vi "IonHeating.vi"(0 "Rotating Wall Parameters":T1={"Start Frequency"=20000.0, "Stop Frequency"=20000.0, "Sweep Time"=0.0, "Amplitude"=1.5, "Phase (ch.1)"=0.001, "Phase (Ch.2)"=90.0} {"Sweep Time" format="%.4f"; "Phase (Ch.2)" min=-1800.0 max=1800.0 step=0.1 format="%.3f"; "Phase (ch.1)" min=-1800.0 max=1800.0 step=0.1 format="%.3f"; "Stop Frequency" format="%#.5p"; "Start Frequency" format="%#.5p"; "Amplitude" min=0.0 max=4.0 format="%.3f"}, 1 "On/Off":bool, 2 "VISAsession":refnum<visa-resource-name>="wavefactoryU10") -> ()   [LabVIEW 2018]
panel:
  out "x-y 5":u32=300
  out "x-y 4":u32=100
  out "x-y 3":u32=901
  out "x-y 2":u32=800
  out "x-y":u32=600
  out "millisecond timer value":u32=88672931
  out "error out":errorcluster caption="Error OUT"
  # "Turn-on\nTimes (ms)"
  # "Turn-off\nTimes (ms)"
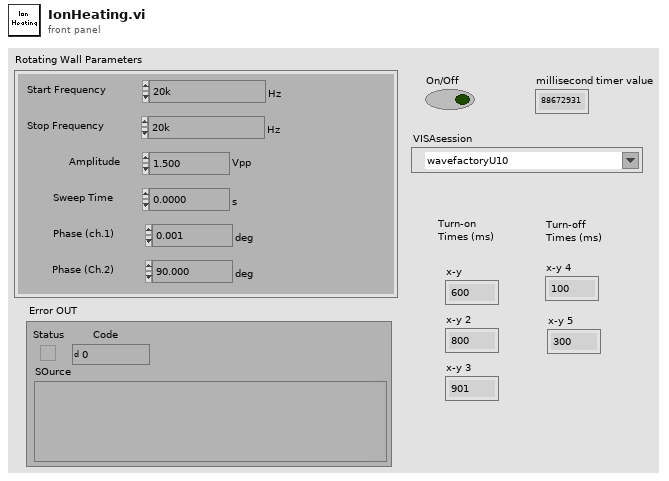
[diagram p1: front panel]
types:
  T1 = cluster{"Start Frequency":dbl, "Stop Frequency":dbl, "Sweep Time":dbl, "Amplitude":dbl, "Phase (ch.1)":dbl, "Phase (Ch.2)":dbl}
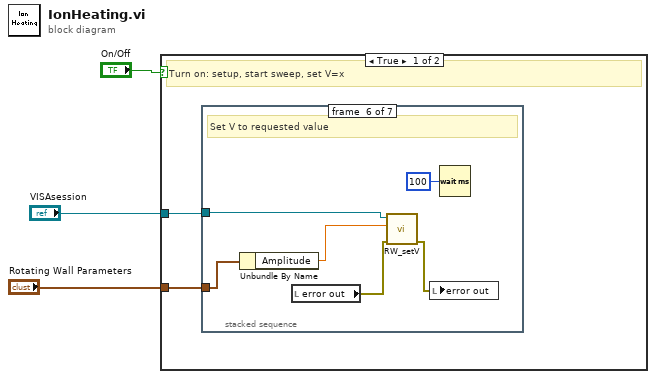
[diagram p0: block diagram]
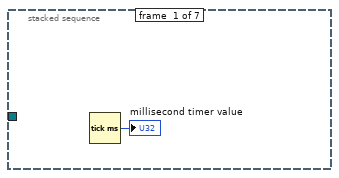
[diagram p2: hidden frame]
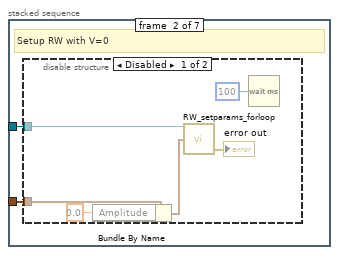
[diagram p3: hidden frame]
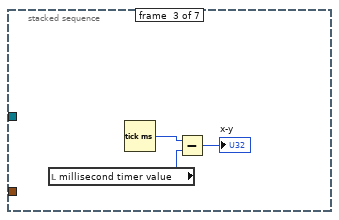
[diagram p5: hidden frame]
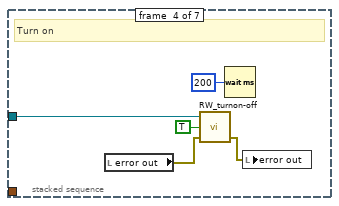
[diagram p6: hidden frame]
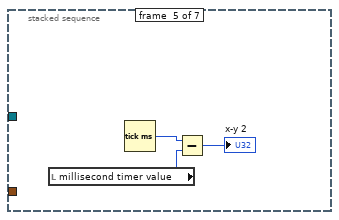
[diagram p7: hidden frame]
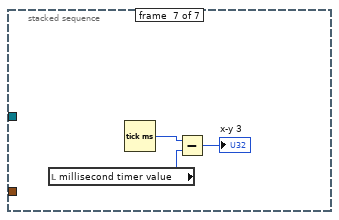
[diagram p8: hidden frame]
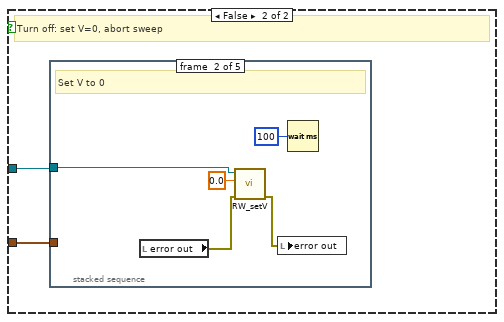
[diagram p9: hidden frame]
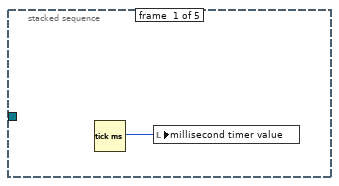
[diagram p10: hidden frame]
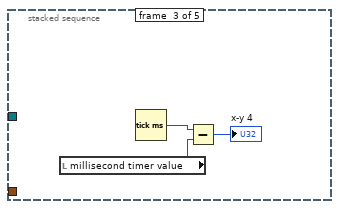
[diagram p11: hidden frame]
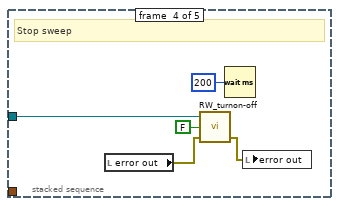
[diagram p12: hidden frame]
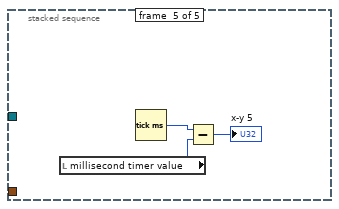
[diagram p13: hidden frame]
diagram:
  n1 = case shown="True" "On/Off" {
    tunnel: "Rotating Wall Parameters" -> [w5 w36]
    tunnel: "VISAsession" -> [w4 w35]
    frame True {
      # "Turn on: setup, start sweep, set V=x"
      n2 = stacked-sequence {
        tunnel: w4 -> [_ w8 _ w21 _ w31 _]
        tunnel: w5 -> [_ w7 _ _ _ w30 _]
        frame #0 {
          n3 = Tick Count (ms)() -> (millisecond timer value=→"millisecond timer value":u32)
        }
        frame #1 {
          # "Setup RW with V=0"
          n4 = disable-structure shown="Disabled" {
            disable-tunnel: w8 -> [w14 _]
            disable-tunnel: w7 -> [w10 _]
            frame Disabled {
              n5 = Bundle By Name(cluster=w10, "Amplitude"=0.0) -> (w9:T1)
              n6 = call "RW_setparams_forloop.vi"("Rotating Wall Parameters"=w9, "VISAsession"=w14) -> ("error out"=→"error out":errorcluster)  [unwired: 2 in, 1 out]
              n7 = Wait (ms)(milliseconds to wait=u32 100) -> ()  [unwired: 1 out]
            }
            frame Enabled {
            }
          }
        }
        frame #2 {
          n8 = local read "millisecond timer value"() -> (w16:u32)
          n9 = Tick Count (ms)() -> (millisecond timer value=w17:u32)
          n10 = Subtract(x=w17, y=w16) -> (x-y=→"x-y":u32)
        }
        frame #3 {
          # "Turn on"
          n11 = local read "error out"() -> (w20:errorcluster)
          n12 = call "RW_turnon-off.vi"("error in (no error)"=w20, "On/Off"=TRUE, "VISAsession"=w21) -> ("error out"=w19:errorcluster)  [unwired: 1 in, 1 out]
          n13 = Wait (ms)(milliseconds to wait=u32 200) -> ()  [unwired: 1 out]
          n14 = local write "error out"(w19) -> ()
        }
        frame #4 {
          n15 = local read "millisecond timer value"() -> (w24:u32)
          n16 = Tick Count (ms)() -> (millisecond timer value=w25:u32)
          n17 = Subtract(x=w25, y=w24) -> (x-y=→"x-y 2":u32)
        }
        frame #5 {
          # "Set V to requested value"
          n18 = Unbundle By Name(w30) -> ("Amplitude"=w27:dbl)
          n19 = local read "error out"() -> (w29:errorcluster)
          n20 = call "RW_setV.vi"("error in (no error)"=w29, "voltage"=w27, "VISAsession"=w31) -> ("error out"=w28:errorcluster)  [unwired: 8 in]
          n21 = local write "error out"(w28) -> ()
          n22 = Wait (ms)(milliseconds to wait=u32 100) -> ()  [unwired: 1 out]
        }
        frame #6 {
          n23 = local read "millisecond timer value"() -> (w33:u32)
          n24 = Tick Count (ms)() -> (millisecond timer value=w34:u32)
          n25 = Subtract(x=w34, y=w33) -> (x-y=→"x-y 3":u32)
        }
      }
    }
    frame False {
      # "Turn off: set V=0, abort sweep"
      n26 = stacked-sequence {
        tunnel: w35 -> [_ w42 _ w49 _]
        tunnel: w36 -> [_ _ _ _ _]
        frame #0 {
          n27 = Tick Count (ms)() -> (millisecond timer value=w37:u32)
          n28 = local write "millisecond timer value"(w37) -> ()
        }
        frame #1 {
          # "Set V to 0"
          n29 = local read "error out"() -> (w41:errorcluster)
          n30 = call "RW_setV.vi"("error in (no error)"=w41, "voltage"=0.0, "VISAsession"=w42) -> ("error out"=w40:errorcluster)  [unwired: 8 in]
          n31 = local write "error out"(w40) -> ()
          n32 = Wait (ms)(milliseconds to wait=u32 100) -> ()  [unwired: 1 out]
        }
        frame #2 {
          n33 = local read "millisecond timer value"() -> (w44:u32)
          n34 = Tick Count (ms)() -> (millisecond timer value=w45:u32)
          n35 = Subtract(x=w45, y=w44) -> (x-y=→"x-y 4":u32)
        }
        frame #3 {
          # "Stop sweep"
          n36 = local read "error out"() -> (w48:errorcluster)
          n37 = call "RW_turnon-off.vi"("error in (no error)"=w48, "On/Off"=FALSE, "VISAsession"=w49) -> ("error out"=w47:errorcluster)  [unwired: 1 in, 1 out]
          n38 = Wait (ms)(milliseconds to wait=u32 200) -> ()  [unwired: 1 out]
          n39 = local write "error out"(w47) -> ()
        }
        frame #4 {
          n40 = local read "millisecond timer value"() -> (w52:u32)
          n41 = Tick Count (ms)() -> (millisecond timer value=w53:u32)
          n42 = Subtract(x=w53, y=w52) -> (x-y=→"x-y 5":u32)
        }
      }
    }
  }
